vi "GageDeepAcquisition.vi"() -> ()   [LabVIEW 2015]
panel:
  in  "Trigger":T1={"Slope"=0, "Level"=0, "Source"=0, "External Range"=2000, "External Coupling"=0, "External"=FALSE, "Disable"=FALSE, "External Impedance"=1} {"External Impedance" items=["50 Ohm", "HiZ"]; "External Coupling" items=["DC", "AC"]; "External Range" min=2000 max=10000 step=8000; "Slope" items=["Rising", "Falling"]; "Level" min=-100 max=100; "Source" min=0 max=64 step=1}
  in  "stop":bool
  in  "Page Size":dbl=32768.0 min=4096.0 step=4096.0
  out "Status":string
  in  "Channels":T2(array[cluster])=[{"Coupling"=0, "Differential Input"=FALSE, "Direct-to-ADC"=FALSE, "Range"=2000, "Impedance"=50, "DC Offset"=0, "Filter"=0}] {"Impedance" min=50 max=1000000 step=999950; "Coupling" items=["DC", "AC"]}
  in  "Acquisition":T3={"Sample Rate"=100000000.0, "Mode"=0, "Depth"=262144.0, "Segment Size"=262144.0, "Trigger Timeout"=1000000.0, "Trigger Holdoff"=0.0, "Trigger Delay"=0.0, "Clock mode"=enum."Internal"} {"Segment Size" min=256.0 step=128.0; "Trigger Delay" min=0.0 step=128.0; "Trigger Holdoff" min=0.0 step=128.0; "Depth" min=256.0 step=128.0; "Mode" items=["Single", "Dual", "Quad", "Octal"]}
  in  "Page":i32=1 min=1 max=8 step=1
  out "System Name":string
  out "Channel Count":u16
  out "Board Count":u16
  in  "Length":dbl=262144.0 min=128.0 max=261120.0
  in  "Start Point":dbl min=1024.0 max=262016.0
  out "Waveform Graph":cluster{dbl, dbl, "Data in Volts":dbl[][]}(graph) caption="Page 1  of  8"
  out "System Count":i32
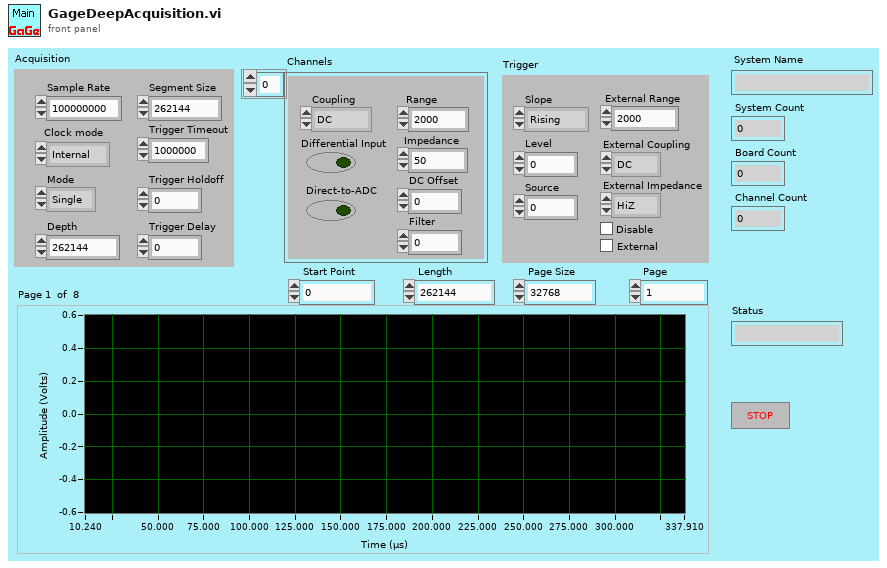
[diagram p1: front panel]
types:
  T1 = cluster{"Slope":u16, "Level":i32, "Source":i32, "External Range":u32, "External Coupling":u16, "External":bool, "Disable":bool, "External Impedance":u16}
  T2 = cluster{"Coupling":u16, "Differential Input":bool, "Direct-to-ADC":bool, "Range":u32, "Impedance":u32, "DC Offset":i32, "Filter":i32}[]
  T3 = cluster{"Sample Rate":dbl, "Mode":u16, "Depth":dbl, "Segment Size":dbl, "Trigger Timeout":dbl, "Trigger Holdoff":dbl, "Trigger Delay":dbl, "Clock mode":enum16{"Internal", "External", "Reference"}}
  T4 = cluster{"Handle":u32, "Sample size":u32, "Resolution":i32, "Offset":i32, "Channels":u32, "Boards":u32}
  T5 = cluster{"Coupling":u16, "Differential Input":bool, "Direct-to-ADC":bool, "Range":u32, "Impedance":u32, "DC Offset":i32, "Filter":i32}
  T6 = cluster{string, "Differential Input":bool, "Direct-to-ADC":bool, "Range":u32, "Impedance":u32, "DC Offset":i32, "Filter":i32}
  T7 = cluster{"RingText.Text":string, "Level":i32, "Source":i32, "External Range":u32, "RingText.Text":string, "External":bool, "Disable":bool, "RingText.Text":string}
  T8 = cluster{"RingText.Text":string, "Level":i32, "Source":i32, "External Range":u32, "RingText.Text":string, "External":bool, "Disable":bool, "RingText.Text":string}[]
  T9 = cluster{"Sample Rate":dbl, "Clock mode":enum16{"Internal", "External", "Reference"}, "RingText.Text":string, "Depth":dbl, "Segment Size":dbl, "Trigger Timeout":dbl, "Trigger Holdoff":dbl, "Trigger Delay":dbl}
  T10 = cluster{"Handle":u32, "Sample Size":u32, "Resolution":i32, "Offset":i32, "Channels":u32, "Boards":u32}
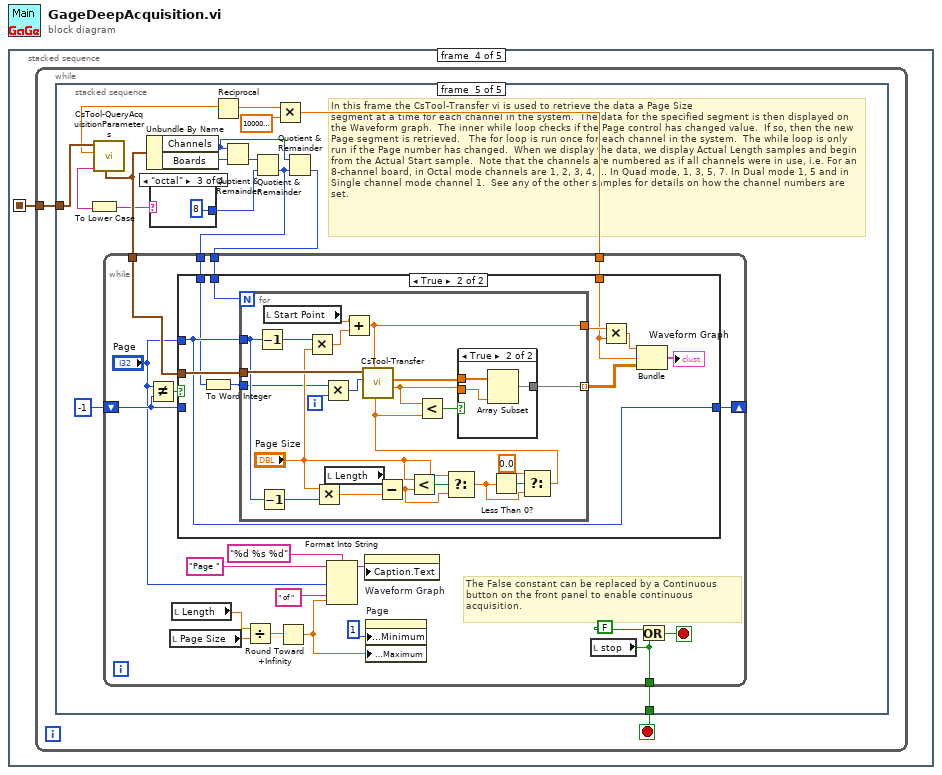
[diagram p0: block diagram]
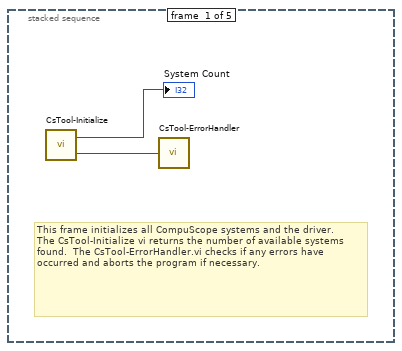
[diagram p2: hidden frame]
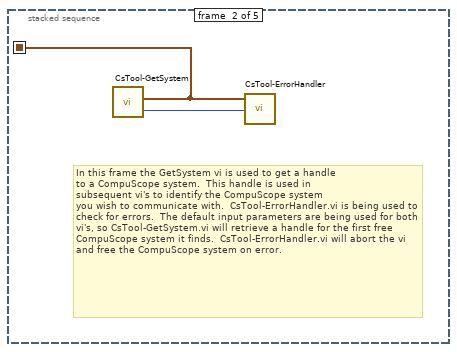
[diagram p3: hidden frame]
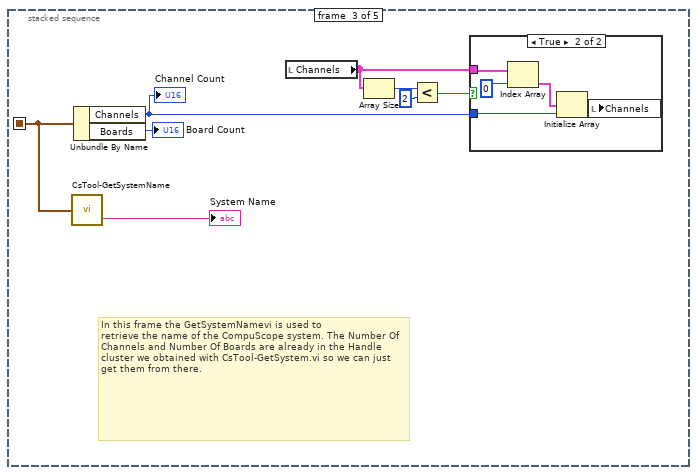
[diagram p4: hidden frame]
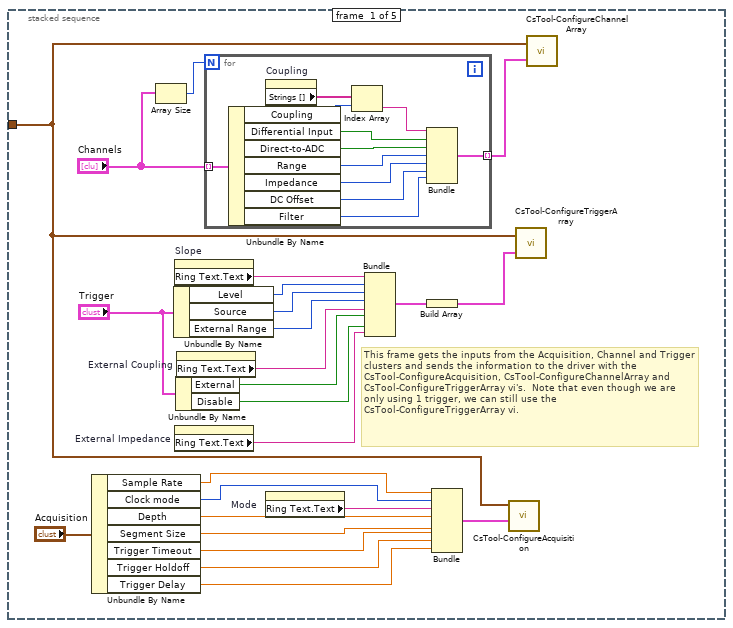
[diagram p6: hidden frame]
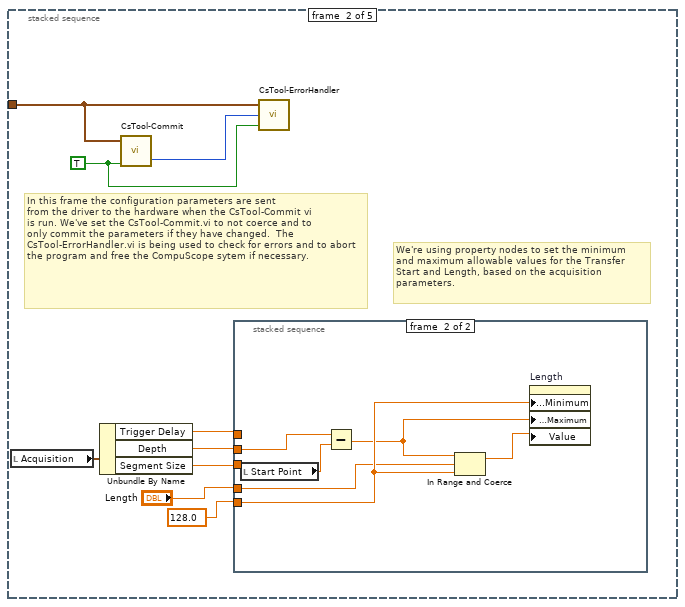
[diagram p7: hidden frame]
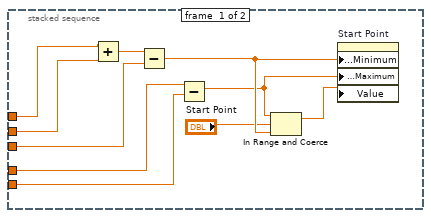
[diagram p8: hidden frame]
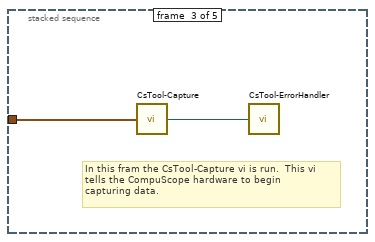
[diagram p9: hidden frame]
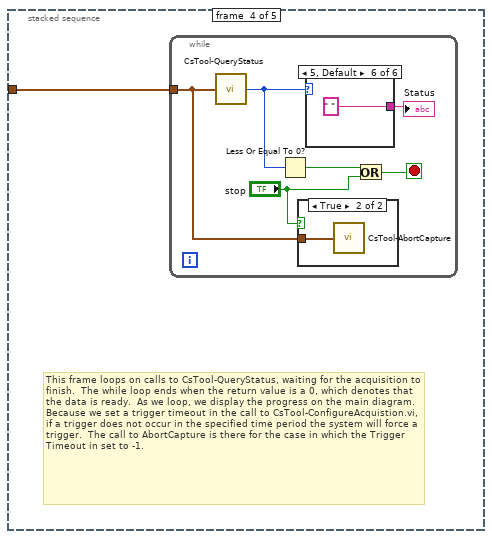
[diagram p10: hidden frame]
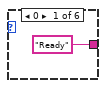
[diagram p12: hidden frame]
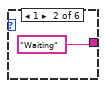
[diagram p13: hidden frame]
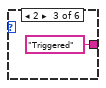
[diagram p14: hidden frame]
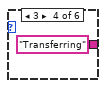
[diagram p15: hidden frame]
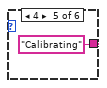
[diagram p16: hidden frame]
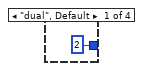
[diagram p17: hidden frame]
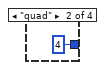
[diagram p18: hidden frame]
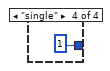
[diagram p19: hidden frame]
diagram:
  n1 = stacked-sequence {
    seq-local: [_ w3 _ _ _] -> [_ _ w11 w18 w176]
    frame #0 {
      # "This frame initializes all CompuScope systems and the driver.\nThe CsTool-Initialize vi returns the number of available systems found.  The CsTool-ErrorHandler.vi checks if any errors have occurred and aborts the program if necessary."
      n2 = call <userlib>:"CsTool-Initialize.vi"() -> ("Error Code"=w2:i32, "Number Of Systems"=→"System Count":i32)
      n3 = call <userlib>:"CsTool-ErrorHandler.vi"("Error Code"=w2) -> ()  [unwired: 2 in, 1 out]
    }
    frame #1 {
      # "In this frame the GetSystem vi is used to get a handle \nto a CompuScope system.  This handle is used in \nsubsequent vi's to identify the CompuScope system \nyou wish to communicate with.  CsTool-ErrorHandler.vi is being used to check for errors.  The default input parameters are being used for both vi's, so CsTool-GetSystem.vi will retrieve a handle for the first free CompuScope system it finds.  CsTool-ErrorHandler.vi will abort the vi and free the CompuScope system on error."
      n4 = call <userlib>:"CsTool-GetSystem.vi"() -> ("Error Code"=w4:i32, "Handle Cluster"=w3:T4)  [unwired: 4 in]
      n5 = call <userlib>:"CsTool-ErrorHandler.vi"("Error Code"=w4, "Handle Cluster"=w3) -> ()  [unwired: 1 in, 1 out]
    }
    frame #2 {
      # "In this frame the GetSystemNamevi is used to\nretrieve the name of the CompuScope system. The Number Of Channels and Number Of Boards are already in the Handle cluster we obtained with CsTool-GetSystem.vi so we can just get them from there."
      n6 = call <userlib>:"CsTool-GetSystemName.vi"("Handle Cluster"=w11) -> ("System Name"=→"System Name":string)  [unwired: 1 out]
      n7 = Unbundle By Name(w11) -> ("Channels"=w10:u32, "Boards"=→"Board Count":u32)
      "Channel Count" <- w10
      n8 = local read "Channels"() -> (w7:T2)
      n9 = Array Size(array=w7) -> (size(s)=w8:i32)
      n10 = Less?(x=w8, y=2) -> (x < y?=w9:bool)
      n11 = case shown="True" w9 {
        tunnel: w7 -> [_ w15]
        tunnel: w10 -> [_ w13]
        frame False {
        }
        frame True {
          n12 = Index Array(array=w15, index=0) -> (element=w14:T5)
          n13 = Initialize Array(w14, w13) -> (w16:T2)
          n14 = local write "Channels"(w16) -> ()
        }
      }
    }
    frame #3 {
      n15 = while {
        tunnel: w18 -> [w20]
        stop <- w19 stop-if-true
        n16 = stacked-sequence {
          tunnel: w20 -> [w39 w63 w82 w84 w112]
          tunnel: [_ _ _ _ w103] -> w19
          frame #0 {
            # "This frame gets the inputs from the Acquisition, Channel and Trigger clusters and sends the information to the driver with the CsTool-ConfigureAcquisition, CsTool-ConfigureChannelArray and CsTool-ConfigureTriggerArray vi's.  Note that even though we are only using 1 trigger, we can still use the CsTool-ConfigureTriggerArray vi."
            n17 = Unbundle By Name("Acquisition") -> ("Sample Rate"=w21:dbl, "Clock mode"=w22:enum16{"Internal", "External", "Reference"}, "Depth"=w45:dbl, "Segment Size"=w28:dbl, "Trigger Timeout"=w27:dbl, "Trigger Holdoff"=w26:dbl, "Trigger Delay"=w25:dbl)
            n18 = Array Size(array="Channels") -> (size(s)=w42:i32)
            n19 = Unbundle By Name("Trigger") -> ("Level"=w37:i32, "Source"=w35:i32, "External Range"=w34:u32)
            n20 = property on="Slope" class="Ring (strict)"() -> ("Ring Text.Text"=w31:string)  [unwired: 2 in, 2 out]
            n21 = property on="External Impedance" class="Ring (strict)"() -> ("Ring Text.Text"=w29:string)  [unwired: 2 in, 2 out]
            n22 = Unbundle By Name("Trigger") -> ("External"=w36:bool, "Disable"=w33:bool)
            n23 = property on="External Coupling" class="Ring (strict)"() -> ("Ring Text.Text"=w30:string)  [unwired: 2 in, 2 out]
            n24 = for {
              N: w42 -> [_]
              tunnel: "Channels" -> [w52] mode=indexing
              tunnel: [w53] -> w40 mode=indexing
              n25 = Unbundle By Name(w52) -> ("Coupling"=w56:u16, "Differential Input"=w51:bool, "Direct-to-ADC"=w50:bool, "Range"=w49:u32, "Impedance"=w48:u32, "DC Offset"=w47:i32, "Filter"=w46:i32)
              n26 = property on="Coupling" class="Ring (strict)"() -> ("Strings []"=w55:string[])  [unwired: 2 in, 2 out]
              n27 = Index Array(array=w55, index=w56) -> (element=w54:string)
              n28 = Bundle(w54, "Differential Input"=w51, "Direct-to-ADC"=w50, "Range"=w49, "Impedance"=w48, "DC Offset"=w47, "Filter"=w46) -> (w53:T6)  [unwired: 1 in]
            }
            n29 = property on="Mode" class="Ring (strict)"() -> ("Ring Text.Text"=w44:string)  [unwired: 2 in, 2 out]
            n30 = Bundle("RingText.Text"=w31, "Level"=w37, "Source"=w35, "External Range"=w34, "RingText.Text"=w30, "External"=w36, "Disable"=w33, "RingText.Text"=w29) -> (w24:T7)  [unwired: 1 in]
            n31 = Build Array(w24) -> (w23:T8)
            n32 = Bundle("Sample Rate"=w21, "Clock mode"=w22, "RingText.Text"=w44, "Depth"=w45, "Segment Size"=w28, "Trigger Timeout"=w27, "Trigger Holdoff"=w26, "Trigger Delay"=w25) -> (w43:T9)  [unwired: 1 in]
            n33 = call <userlib>:"CsTool-ConfigureAcquisition.vi"("Handle Cluster"=w39, "Acquisition"=w43) -> ()  [unwired: 3 in, 1 out]
            n34 = call <userlib>:"CsTool-ConfigureTriggerArray.vi"("Triggers"=w23, "Handle Cluster"=w39) -> ()  [unwired: 1 out]
            n35 = call <userlib>:"CsTool-ConfigureChannelArray.vi"("Channels"=w40, "Handle Cluster"=w39) -> ()  [unwired: 1 out]
          }
          frame #1 {
            w64 = TRUE
            # "We're using property nodes to set the minimum\nand maximum allowable values for the Transfer \nStart and Length, based on the acquisition \nparameters."
            # "In this frame the configuration parameters are sent\nfrom the driver to the hardware when the CsTool-Commit vi \nis run. We've set the CsTool-Commit.vi to not coerce and to\nonly commit the parameters if they have changed.  The CsTool-ErrorHandler.vi is being used to check for errors and to abort the program and free the CompuScope sytem if necessary."
            n36 = local read "Acquisition"() -> (w61:T3)
            n37 = Unbundle By Name(w61) -> ("Trigger Delay"=w60:dbl, "Depth"=w62:dbl, "Segment Size"=w59:dbl)
            n38 = call <userlib>:"CsTool-Commit.vi"("OnlyOnChange (t)"=w64, "Handle Cluster"=w63) -> ("Error Code"=w65:i32)  [unwired: 1 in, 1 out]
            n39 = stacked-sequence {
              tunnel: w60 -> [w75 _]
              tunnel: w62 -> [w74 w78]
              tunnel: w59 -> [w72 _]
              tunnel: "Length" -> [w71 w80]
              tunnel: 128.0 -> [w70 w81]
              frame #0 {
                n40 = Add(x=w75, y=w74) -> (x+y=w73:dbl)
                n41 = Subtract(x=w73, y=w72) -> (x-y=w69:dbl)
                n42 = Subtract(x=w71, y=w70) -> (x-y=w68:dbl)
                n43 = In Range and Coerce(upper limit=w68, x="Start Point", lower limit=w69) -> (coerced(x)=w67:dbl)  [unwired: 1 out]
                n44 = property on="Start Point" class="DigNum (strict)"("Data Entry Limits:Minimum"=w69, "Data Entry Limits:Maximum"=w68, "Value"=w67) -> ()  [unwired: 2 in, 2 out]
              }
              frame #1 {
                n45 = local read "Start Point"() -> (w77:dbl)
                n46 = Subtract(x=w78, y=w77) -> (x-y=w76:dbl)
                n47 = In Range and Coerce(upper limit=w76, x=w80, lower limit=w81) -> (coerced(x)=w79:dbl)  [unwired: 1 out]
                n48 = property on="Length" class="DigNum (strict)"("Data Entry Limits:Minimum"=w81, "Data Entry Limits:Maximum"=w76, "Value"=w79) -> ()  [unwired: 2 in, 2 out]
              }
            }
            n49 = call <userlib>:"CsTool-ErrorHandler.vi"("StopOnError (true)"=w64, "Error Code"=w65, "Handle Cluster"=w63) -> ()  [unwired: 1 out]
          }
          frame #2 {
            # "In this fram the CsTool-Capture vi is run.  This vi\ntells the CompuScope hardware to begin\ncapturing data."
            n50 = call <userlib>:"CsTool-Capture.vi"("Handle Cluster"=w82) -> ("Error Code"=w83:i32)
            n51 = call <userlib>:"CsTool-ErrorHandler.vi"("Error Code"=w83) -> ()  [unwired: 2 in, 1 out]
          }
          frame #3 {
            # "This frame loops on calls to CsTool-QueryStatus, waiting for the acquisition to finish.  The while loop ends when the return value is a 0, which denotes that the data is ready.  As we loop, we display the progress on the main diagram.  Because we set a trigger timeout in the call to CsTool-ConfigureAcquistion.vi, if a trigger does not occur in the specified time period the system will force a trigger.  The call to AbortCapture is there for the case in which the Trigger Timeout in set to -1."
            n52 = while {
              tunnel: w84 -> [w86]
              stop <- w87 stop-if-true
              n53 = call <userlib>:"CsTool-QueryStatus.vi"("Handle Cluster"=w86) -> ("Status"=w90:i32)
              n54 = Less Or Equal To 0?(x=w90) -> (x <= 0?=w88:bool)
              n55 = case shown="True" "stop" {
                tunnel: w86 -> [_ w91]
                frame False {
                }
                frame True {
                  n56 = call <userlib>:"CsTool-AbortCapture.vi"("Handle Cluster"=w91) -> ()  [unwired: 1 out]
                }
              }
              n57 = case shown="5, Default" w90 {
                tunnel: ["Ready" "Waiting" "Triggered" "Transferring" "Calibrating" " "] -> w89
                frame 0 {
                }
                frame 1 {
                }
                frame 2 {
                }
                frame 3 {
                }
                frame 4 {
                }
                frame 5, Default {
                }
              }
              "Status" <- w89
              n58 = Or(x=w88, y="stop") -> (x .or. y?=w87:bool)
            }
          }
          frame #4 {
            # "In this frame the CsTool-Transfer vi is used to retrieve the data a Page Size \nsegment at a time for each channel in the system.  The data for the specified segment is then displayed on the Waveform graph.  The inner while loop checks if the Page control has changed value.  If so, then the new Page segment is retrieved.   The for loop is run once for each channel in the system.  The while loop is only run if the Page number has changed.  When we display the data, we display Actual Length samples and begin from the Actual Start sample.  Note that the channels are numbered as if all channels were in use, i.e. For an 8-channel board, in Octal mode channels are 1, 2, 3, 4, ... In Quad mode, 1, 3, 5, 7. In Dual mode 1, 5 and in Single channel mode channel 1.  See any of the other samples for details on how the channel numbers are set."
            n59 = call <userlib>:"CsTool-QueryAcquisitionParameters.vi"("Handle Cluster"=w112) -> ("Output Handle Cluster"=w111:T10, "Mode"=w110:string, "Sample Rate"=w101:dbl)  [unwired: 8 out]
            n60 = To Lower Case(string=w110) -> (all lower case string=w109:string)
            n61 = Unbundle By Name(w111) -> ("Channels"=w106:u32, "Boards"=w102:u32)
            n62 = case shown="\"octal\"" w109 {
              tunnel: [2 4 8 1] -> w107
              frame "dual", Default {
              }
              frame "quad" {
              }
              frame "octal" {
              }
              frame "single" {
              }
            }
            n63 = Reciprocal(x=w101) -> (1/x=w100:dbl)
            n64 = Quotient & Remainder(x=w106, y=w102) -> (floor(x/y)=w108:u32)  [unwired: 1 out]
            n65 = Quotient & Remainder(x=w108, y=w107) -> (floor(x/y)=w105:u32)  [unwired: 1 out]
            n66 = Multiply(x=w100, y=1000000.0) -> (x*y=w98:dbl)
            n67 = Quotient & Remainder(x=w106, y=w105) -> (floor(x/y)=w104:u32)  [unwired: 1 out]
            n68 = while {
              shift-right: [w136] -> _
              shift-left: -1 -> [w135]
              tunnel: w111 -> [w122]
              tunnel: w98 -> [w128]
              tunnel: w104 -> [w127]
              tunnel: w105 -> [w126]
              tunnel: [w123] -> w103
              stop <- w134 stop-if-true
              # "The False constant can be replaced by a Continuous\nbutton on the front panel to enable continuous\nacquisition."
              n69 = Not Equal?(x="Page", y=w135) -> (x != y?=w137:bool)
              n70 = local read "Page Size"() -> (w125:dbl)
              n71 = local read "Length"() -> (w118:dbl)
              n72 = case shown="True" w137 {
                tunnel: "Page" -> [_ w143]
                tunnel: [w138 w143] -> w136
                tunnel: w135 -> [w138 _]
                tunnel: w122 -> [_ w147]
                tunnel: w128 -> [_ w139]
                tunnel: w127 -> [_ w142]
                tunnel: w126 -> [_ w141]
                frame False {
                }
                frame True {
                  n73 = To Word Integer(number=w141) -> ()  [unwired: 1 out]
                  n74 = for {
                    N: w142 -> [_]
                    tunnel: [w167] -> w145 mode=indexing
                    tunnel: w147 -> [w170]
                    tunnel: [w149] -> w140
                    tunnel: w143 -> [w154]
                    tunnel: w141 -> [w151]
                    i -> [w152]
                    n75 = Decrement(x=w154) -> (x-1=w166:i32)
                    n76 = Decrement(x=w154) -> (x-1=w157:i32)
                    n77 = local read "Start Point"() -> (w148:dbl)
                    n78 = Multiply(x=w166, y="Page Size") -> (x*y=w165:dbl)
                    n79 = Multiply(x="Page Size", y=w157) -> (x*y=w163:dbl)
                    n80 = Multiply(x=w151, y=w152) -> (x*y=w150:u32)
                    n81 = local read "Length"() -> (w164:dbl)
                    n82 = Add(x=w148, y=w165) -> (x+y=w149:dbl)
                    n83 = Subtract(x=w164, y=w163) -> (x-y=w161:dbl)
                    n84 = Less?(x="Page Size", y=w161) -> (x < y?=w162:bool)
                    n85 = Select(t="Page Size", s=w162, f=w161) -> (s? t:f=w158:dbl)
                    n86 = Less Than 0?(x=w158) -> (x < 0?=w160:bool)
                    n87 = Select(t=0.0, s=w160, f=w158) -> (s? t:f=w155:dbl)
                    n88 = call <userlib>:"CsTool-Transfer.vi"("Length (4096)"=w155, "Start (0)"=w149, "Channel (0)"=w150, "Handle Cluster"=w170) -> ("Actual Length"=w153:dbl, "Data in Volts"=w168:dbl[])  [unwired: 2 in, 2 out]
                    n89 = Less?(x=w153, y=w155) -> (x < y?=w169:bool)
                    n90 = case shown="True" w169 {
                      tunnel: w168 -> [w171 w174]
                      tunnel: [w171 w173] -> w167
                      tunnel: w153 -> [_ w172]
                      frame False {
                      }
                      frame True {
                        n91 = Array Subset(array=w174, length=w172) -> (w173:dbl[])  [unwired: 1 in]
                      }
                    }
                  }
                  n92 = Multiply(x=w140, y=w139) -> (x*y=w146:dbl)
                  n93 = Bundle(w146, w139, "Data in Volts"=w145) -> (→"Waveform Graph":cluster{dbl, dbl, "Data in Volts":dbl[][]})  [unwired: 1 in]
                }
              }
              n94 = Divide(x=w118, y=w125) -> (x/y=w124:dbl)
              n95 = Round Toward +Infinity(x=w124) -> (ceil(x): smallest int >= x=w120:dbl)
              n96 = Format Into String(format string="%d %s %d", initial string="Page ", "Page", " of ", w120) -> (resulting string=w131:string)  [unwired: 1 in, 1 out]
              n97 = property on="Waveform Graph" class="WFGraph (strict)"("Caption.Text"=w131) -> ()  [unwired: 2 in, 2 out]
              n98 = property on="Page" class="DigNum (strict)"("Data Entry Limits:Minimum"=1, "Data Entry Limits:Maximum"=w120) -> ()  [unwired: 2 in, 2 out]
              n99 = local read "stop"() -> (w123:bool)
              n100 = Or(x=FALSE, y=w123) -> (x .or. y?=w134:bool)
            }
          }
        }
      }
    }
    frame #4 {
      # "We set the Stop button (actually it's local variable) to False here so when the vi stops the Stop button will not stay depressed."
      # "In this frame, which is reached when the Stop\nis pressed, the CompuScope system is freed by\nrunning the CsTool-FreeSystem vi.  This frees \nany resources used by the system and makes \nit available for another program to use."
      n101 = call "CsTool-FreeSystem.vi"("Handle Cluster"=w176) -> ()  [unwired: 1 out]
      n102 = local write "stop"(FALSE) -> ()
    }
  }
